vi "Write Card Cluster.vi"(10 "Card Cluster":T1, 11 "WT1600 in":refnum<class "WT1600.lvclass">) -> (3 "WT1600 out":refnum<class "WT1600.lvclass">)   [LabVIEW 2013, in "Universal Power Meter.lvlib" / "WT1600.lvlib" / "WT1600.lvclass"]
uses:
  WT1600.lvclass
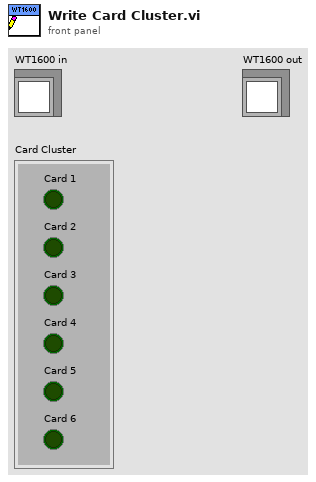
[diagram p1: front panel]
types:
  T1 = cluster{"Card 1":bool, "Card 2":bool, "Card 3":bool, "Card 4":bool, "Card 5":bool, "Card 6":bool}
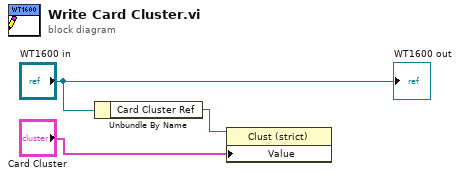
[diagram p0: block diagram]
diagram:
  n1 = Unbundle By Name("WT1600 in") -> ("Card Cluster Ref"=w2:refnum<vi>)
  n2 = property class="Clust (strict)"(reference=w2, "Value"="Card Cluster") -> ()  [unwired: 1 in, 2 out]
  "WT1600 out" <- "WT1600 in"
